vi "Get Row and Colum (SubVI).vi"(8 "Dim":u16=256, 10 "Colum In":u8, 11 "Row In":u8) -> (0 "Last Pixel?":bool, 2 "Colum Out":u8, 3 "Row Out":u8, 4 "Pixel B":u16, 6 "Pixel A":u16)   [LabVIEW 2017, in "SoC IP Library.lvlib"]
uses:
  SoC IP Library.lvlib
  <vilib>/rvi/FXPMathLib/FxpMul/XNode/nifxpmath_Multiplier.xnode
  <vilib>/rvi/FXPMathLib/sim/FxpSim.dll
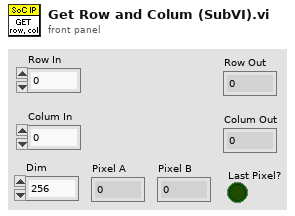
[diagram p1: front panel]
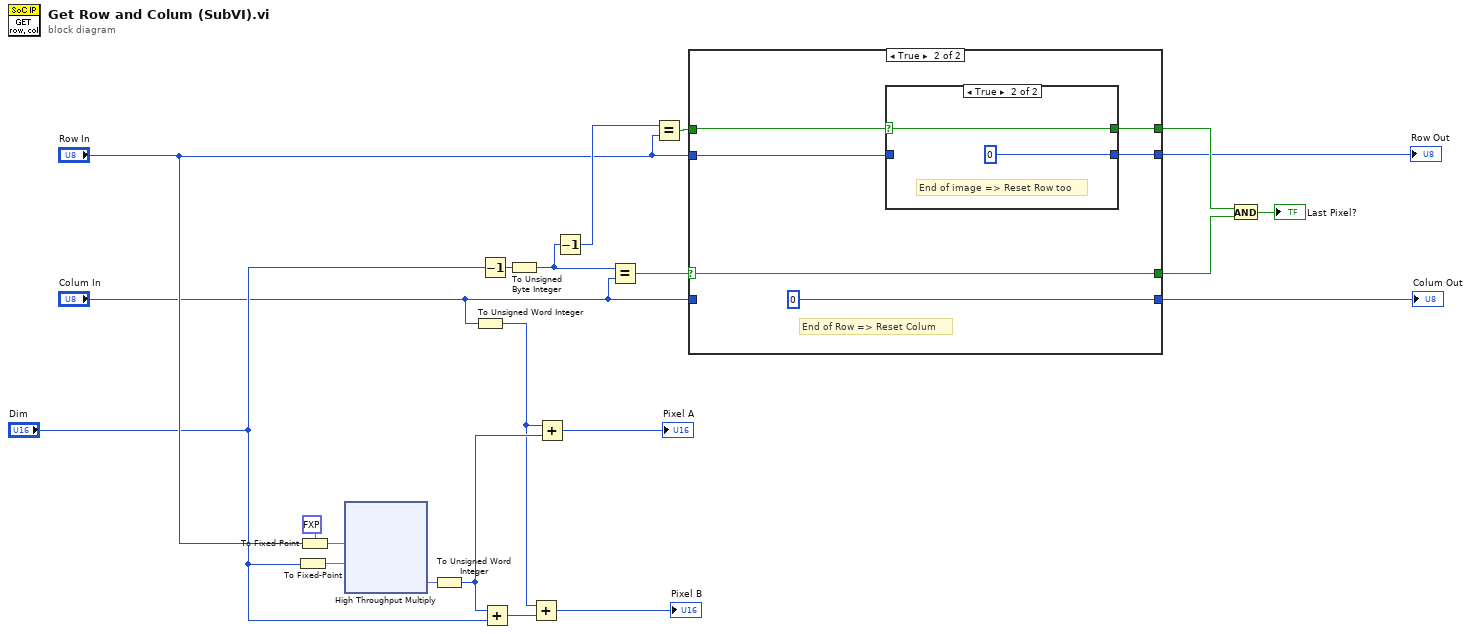
[diagram p0: block diagram]
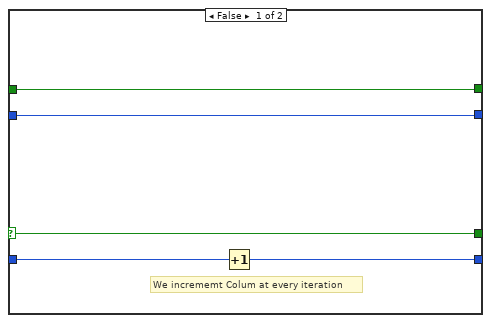
[diagram p2: hidden frame]
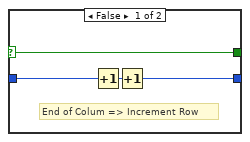
[diagram p3: hidden frame]
diagram:
  n1 = To Fixed-Point(number="Dim") -> (fixed-point=w6:fxp<+,16,16>)  [unwired: 1 in]
  n2 = To Fixed-Point(fixed-point type=fxp<+,8,8> 0.0 ("x"), number="Row In") -> (fixed-point=w8:fxp<+,8,8>)
  n3 = xnode ("High Throughput Multiply")("x"=w8, "y"=w6) -> ("x*y"=w9:fxp<+,16,16>)
  n4 = To Unsigned Word Integer(number=w9) -> (unsigned 16bit integer=w3:u16)
  n5 = To Unsigned Word Integer(number="Colum In") -> (unsigned 16bit integer=w1:u16)
  n6 = Decrement(x="Dim") -> (x-1=w13:u16)
  n7 = Add(x=w3, y="Dim") -> (x+y=w10:u16)
  n8 = To Unsigned Byte Integer(number=w13) -> (unsigned 8bit integer=w4:u8)
  n9 = Add(x=w1, y=w10) -> (x+y=→"Pixel B":u16)
  n10 = Add(x=w1, y=w3) -> (x+y=→"Pixel A":u16)
  n11 = Decrement(x=w4) -> (x-1=w12:u8)
  n12 = Equal?(x=w4, y="Colum In") -> (x = y?=w22:bool)
  n13 = Equal?(x=w12, y="Row In") -> (x = y?=w16:bool)
  n14 = case shown="True" w22 {
    selector: w22 -> [w25 w32]
    tunnel: [w27 u8 0] -> w21
    tunnel: "Colum In" -> [w26 _]
    tunnel: [w25 w32] -> w20
    tunnel: w16 -> [w23 w31]
    tunnel: "Row In" -> [w24 w28]
    tunnel: [w24 w30] -> w14
    tunnel: [w23 w29] -> w15
    frame False {
      # "We incrememt Colum at every iteration"
      n15 = Increment(x=w26) -> (x+1=w27:u8)
    }
    frame True {
      # "End of Row => Reset Colum"
      n16 = case shown="True" w31 {
        selector: w31 -> [w34 w38]
        tunnel: [w35 u8 0] -> w30
        tunnel: w28 -> [w36 _]
        tunnel: [w34 w38] -> w29
        frame False {
          # "End of Colum => Increment Row"
          n17 = Increment(x=w36) -> (x+1=w37:u8)
          n18 = Increment(x=w37) -> (x+1=w35:u8)
        }
        frame True {
          # "End of image => Reset Row too"
        }
      }
    }
  }
  "Row Out" <- w14
  "Colum Out" <- w21
  n19 = And(x=w15, y=w20) -> (x .and. y?=→"Last Pixel?":bool)
